vi "S4GUI.vi"(7 "Tab ObsEng":enum32{"Obs", "CCD modes", "Guider", "Eng"}(tab)) -> ()   [LabVIEW 2018] (continued)
        # "real"
        # "Inicializar nova comunicação, de acordo\n com valor de TCS mode\n\nServer.Write id (T=6 ou F=12)\nTCS.Init"
        # "Parar a comunciação atual\nServer.End"
        n1486 = event-data() -> ("NewVal"=w2535:bool)  [unwired: 1 in, 5 out]
        n1487 = call-dynamic "Read TCS.lvclass.vi"("error in (no error)"=w2545, "S4GUI in"=w2546) -> ("error out"=w2540:errorcluster, "TCS.lvclass"=w2543:refnum<class "TCS.lvclass">, "S4GUI out"=w2544:refnum<class "S4GUI.lvclass">)  [unwired: 7 in]
        n1488 = call-dynamic "End.vi"("error in (no error)"=w2540, "Server in"=w2543) -> ("error out"=w2539:errorcluster, "Server out"=w2542:refnum<class "TCS.lvclass">)  [unwired: 8 in]
        n1489 = Select(t=u32 6, s=w2535, f=u32 12) -> (s? t:f=w2549:u32)
        n1490 = call-dynamic "Write id.vi"("error in (no error)"=w2539, "id"=w2549, "Server in"=w2542) -> ("error out"=w2538:errorcluster, "Server out"=w2541:refnum<class "TCS.lvclass">)  [unwired: 7 in]
        n1491 = call-dynamic "Initialize.vi"("error in (no error)"=w2538, "TCS in"=w2541) -> ("error out"=w2536:errorcluster, "TCS out"=w2537:refnum<class "TCS.lvclass">)  [unwired: 8 in]
        n1492 = call-dynamic "Write TCS.lvclass.vi"("error in (no error)"=w2536, "TCS.lvclass"=w2537, "S4GUI in"=w2544) -> ("error out"=w2533:errorcluster, "S4GUI out"=w2534:refnum<class "S4GUI.lvclass">)  [unwired: 7 in]
      }
      event "enter password": Value Change {
        n1493 = event-data() -> ("NewVal"=w2550:bool)  [unwired: 1 in]
        n1494 = case shown="True" w2550 {
          tunnel: [w2556 w2558] -> w2554
          tunnel: [w2555 w2557] -> w2553
          tunnel: w2552 -> [w2556 w2571]
          tunnel: w2551 -> [w2555 w2570]
          frame False {
          }
          frame True {
            # "Verifica senha de configuração de CCD do Administrador"
            n1495 = Equal?(x="password", y="camerasetup") -> (x = y?=w2568:bool)
            n1496 = call-dynamic "Write mode Adm.vi"("error in (no error)"=w2570, "mode Adm"=w2568, "S4GUI in"=w2571) -> ("error out"=w2559:errorcluster, "S4GUI out"=w2560:refnum<class "S4GUI.lvclass">)  [unwired: 7 in]
            n1497 = call-dynamic "Read mode Adm.vi"("error in (no error)"=w2559, "S4GUI in"=w2560) -> ("error out"=w2566:errorcluster, "mode Adm"=w2563:bool, "S4GUI out"=w2565:refnum<class "S4GUI.lvclass">)  [unwired: 7 in]
            n1498 = Select(t="Eng/Camera tab: password OK clicked successful" ("User Event"), s=w2563, f="Eng/Camera tab: password OK clicked with wrong input" ("User Event")) -> (s? t:f=w2564:string)
            n1499 = call-dynamic "Write User Event.vi"("error in (no error)"=w2566, "User Event"=w2564, "S4GUI in"=w2565) -> ("error out"=w2557:errorcluster, "S4GUI out"=w2558:refnum<class "S4GUI.lvclass">)  [unwired: 7 in]
          }
        }
      }
      event "enter password 2": Value Change {
        # "Verificação de senha na aba \"CCD modes\""
        n1500 = event-data() -> ("NewVal"=w2572:bool)  [unwired: 1 in]
        n1501 = case shown="True" w2572 {
          tunnel: [w2578 w2588] -> w2576
          tunnel: [w2577 w2587] -> w2575
          tunnel: w2574 -> [w2578 w2593]
          tunnel: w2573 -> [w2577 w2592]
          frame False {
          }
          frame True {
            # "Verifica senha de configuração de CCD do Administrador"
            n1502 = Equal?(x="password 2", y="ccdmodessetup") -> (x = y?=w2590:bool)
            n1503 = call-dynamic "Write mode Adm.vi"("error in (no error)"=w2592, "mode Adm"=w2590, "S4GUI in"=w2593) -> ("error out"=w2585:errorcluster, "S4GUI out"=w2586:refnum<class "S4GUI.lvclass">)  [unwired: 7 in]
            n1504 = call-dynamic "Read mode Adm.vi"("error in (no error)"=w2585, "S4GUI in"=w2586) -> ("error out"=w2583:errorcluster, "mode Adm"=w2580:bool, "S4GUI out"=w2584:refnum<class "S4GUI.lvclass">)  [unwired: 7 in]
            n1505 = Select(t="CCD mode tab: password OK clicked successful" ("User Event"), s=w2580, f="CCD mode tab: password OK clicked with wrong input" ("User Event")) -> (s? t:f=w2581:string)
            n1506 = call-dynamic "Write User Event.vi"("error in (no error)"=w2583, "User Event"=w2581, "S4GUI in"=w2584) -> ("error out"=w2587:errorcluster, "S4GUI out"=w2588:refnum<class "S4GUI.lvclass">)  [unwired: 7 in]
          }
        }
      }
      event "Tab ObsEng": Value Change {
        n1507 = event-data() -> ("NewVal"=w2594:enum32{"Obs", "CCD modes", "Guider", "Eng"})  [unwired: 1 in]
        n1508 = case shown="Default" w2594 {
          tunnel: [w2608 w2760 w2771] -> w2598
          tunnel: [w2610 w2758 w2769] -> w2597
          tunnel: w2596 -> [w2605 w2766 w2775]
          tunnel: w2595 -> [w2604 w2657 w2770]
          frame "CCD modes" {
            # "Sinaliza que não há requisição de SET CCD mode"
            # "Entrou na aba \"CCD modes\", ajusta para modo usuário normal..."
            n1509 = call-dynamic "Read TabAcqType index.vi"("error in (no error)"=w2604, "S4GUI in"=w2605) -> ("error out"=w2603:errorcluster, "TabAcqType index"=w2601:u32, "S4GUI out"=w2602:refnum<class "S4GUI.lvclass">)  [unwired: 7 in]
            n1510 = case shown="4" w2601 {
              tunnel: w2603 -> [w2640 w2645]
              tunnel: [w2639 w2644] -> w2606
              tunnel: [w2638 w2643] -> w2600
              tunnel: [FALSE ("Visible") TRUE ("Visible")] -> w2599
              frame 0, Default {
                n1511 = local read "Frame Transfer"() -> (w2638:enum16{"OFF", "ON"})
                n1512 = property on="Frame Transfer" class="Enum (strict)"(error in=w2640, "DisabledEnum"=T12."Enabled" ("Disabled")) -> (error out=w2639:errorcluster)  [unwired: 1 in, 1 out]
              }
              frame 4 {
                w2643 = enum16{"OFF", "ON"}."OFF" ("Frame Transfer")
                n1513 = property on="Frame Transfer" class="Enum (strict)"(error in=w2645, "DisabledEnum"=T12."Disabled and Grayed Out" ("Disabled"), "Value"=w2643) -> (error out=w2644:errorcluster)  [unwired: 1 in, 1 out]
              }
            }
            n1514 = property on="FT warning" class="Str"("Caption.Visible"=w2599) -> ()  [unwired: 2 in, 2 out]
            n1515 = call-dynamic "Write mode Adm.vi"("error in (no error)"=w2606, "mode Adm"=FALSE, "S4GUI in"=w2602) -> ("error out"=w2632:errorcluster, "S4GUI out"=w2634:refnum<class "S4GUI.lvclass">)  [unwired: 7 in]
            n1516 = local write "password 2"("" ("password")) -> ()
            n1517 = call-dynamic "Write SET request.vi"("error in (no error)"=w2632, "SET request"=FALSE, "S4GUI in"=w2634) -> ("error out"=w2631:errorcluster, "S4GUI out"=w2633:refnum<class "S4GUI.lvclass">)  [unwired: 7 in]
            n1518 = disable-structure shown="Disabled" {
              frame Disabled {
                n1519 = flat-sequence {
                  tunnel: _ -> [w2653]
                  tunnel: [w2653] -> _
                  frame #0 {
                    n1520 = local read "AQM"() -> (w2650:T4)
                    n1521 = Less Or Equal?(x=w2650, y=T4."NORMAL FAINT: Conventional; 1 MHz; Gain 2") -> (x <= y?=w2649:bool)
                    n1522 = Select(t=w2650, s=w2649, f=T4."SLOW BRIGHT: Conventional; 0.1 MHz; Gain 1" ("y")) -> (s? t:f=w2651:T4)
                    n1523 = local write "EM Gain"(u16 2 ("EM Gain")) -> ()
                    n1524 = local write "AQM"(w2651) -> ()
                  }
                }
              }
              frame Enabled {
              }
            }
            n1525 = flat-sequence {
              tunnel: w2631 -> [w2656]
              tunnel: [w2656] -> w2617
              tunnel: [w2655] -> w2614
              tunnel: [w2654] -> w2615
              frame #0 {
                w2654 = u16 2 ("EM Gain")
                w2655 = T4."NORMAL FAINT: Conventional; 1 MHz; Gain 2" ("AQM")
                n1526 = local write "EM Gain"(w2654) -> ()
                n1527 = local write "AQM"(w2655) -> ()
              }
            }
            n1528 = call-dynamic "Read CCD mode.vi"("error in (no error)"=w2617, "S4GUI in"=w2633) -> ("error out"=w2622:errorcluster, "CCD mode"=w2620:T30, "S4GUI out"=w2619:refnum<class "S4GUI.lvclass">)  [unwired: 7 in]
            n1529 = local read "SZM"() -> (w2616:T3)
            n1530 = Bundle By Name(cluster=w2620, "FTM"=w2600, "SZM"=w2616, "EM gain"=w2615, "AQM"=w2614) -> (w2621:T30)
            n1531 = call-dynamic "Write CCD mode.vi"("error in (no error)"=w2622, "CCD mode"=w2621, "S4GUI in"=w2619) -> ("error out"=w2624:errorcluster, "S4GUI out"=w2623:refnum<class "S4GUI.lvclass">)  [unwired: 7 in]
            n1532 = call-dynamic "LoadCCDmode.vi"("error in (no error)"=w2624, "S4GUI in"=w2623) -> ("error out"=w2626:errorcluster, "S4GUI out"=w2625:refnum<class "S4GUI.lvclass">)  [unwired: 8 in]
            n1533 = call-dynamic "Read Parameters CCD modes.vi"("error in (no error)"=w2626, "S4GUI in"=w2625) -> ("error out"=w2629:errorcluster, "Parameters CCD modes"=w2618:T5, "S4GUI out"=w2627:refnum<class "S4GUI.lvclass">)  [unwired: 7 in]
            n1534 = local write "Parameters CCD modes"(w2618) -> ()
            n1535 = call-dynamic "Read InfoCCDmode.vi"("error in (no error)"=w2629, "S4GUI in"=w2627) -> ("error out"=w2612:errorcluster, "InfoCCDmode"=w2628:T2, "S4GUI out"=w2613:refnum<class "S4GUI.lvclass">)  [unwired: 7 in]
            n1536 = local write "InfoCCDmode"(w2628) -> ()
            n1537 = call-dynamic "CalcTemp.vi"("error in (no error)"=w2612, "S4GUI in"=w2613) -> ("error out"=w2611:errorcluster, "S4GUI out"=w2609:refnum<class "S4GUI.lvclass">)  [unwired: 8 in]
            n1538 = call-dynamic "Read Prev Temp.vi"("error in (no error)"=w2611, "S4GUI in"=w2609) -> ("error out"=w2610:errorcluster, "Prev Temp"=w2607:dbl, "S4GUI out"=w2608:refnum<class "S4GUI.lvclass">)  [unwired: 7 in]
            n1539 = local write "Preview Temp."(w2607) -> ()
          }
          frame "Eng" {
            w2764 = T12."Disabled and Grayed Out" ("Disabled")
            # "Desabilita os botões SET."
            # "Entrou na aba  \"Eng\", ajusta para modo usuário normal..."
            n1540 = local write "password"("" ("password")) -> ()
            n1541 = call-dynamic "Write mode Adm.vi"("error in (no error)"=w2657, "mode Adm"=FALSE, "S4GUI in"=w2766) -> ("error out"=w2759:errorcluster, "S4GUI out"=w2762:refnum<class "S4GUI.lvclass">)  [unwired: 7 in]
            n1542 = property on="Set from Input ch1" class="Bool"("DisabledEnum"=w2764) -> ()  [unwired: 2 in, 2 out]
            n1543 = property on="Set from Input ch3" class="Bool"("DisabledEnum"=w2764) -> ()  [unwired: 2 in, 2 out]
            n1544 = property on="Set from Input ch2" class="Bool"("DisabledEnum"=w2764) -> ()  [unwired: 2 in, 2 out]
            n1545 = property on="Set from Input ch4" class="Bool"("DisabledEnum"=w2764) -> ()  [unwired: 2 in, 2 out]
            n1546 = local read "TARGET NAME WPSEL"() -> (w2715:enum16{"NONE", "OFF", "L/2", "L/4"})
            n1547 = call "Read Instrument.lvclass.vi"("error in (no error)"=w2759, "S4ACS_GUI in"=w2762) -> ("error out"=w2740:errorcluster, "Instrument.lvclass"=w2757:refnum<class "Instrument.lvclass">, "S4ACS_GUI out"=w2761:refnum<class "S4GUI.lvclass">)  [unwired: 7 in]
            n1548 = local read "TARGET NAME CALW"() -> (w2705:T9)
            n1549 = property on="TARGET NAME WPSEL" class="Enum (strict)"() -> ("RingText.Text"=w2713:string)  [unwired: 2 in, 2 out]
            n1550 = call "Read WPSEL.vi"("error in (no error)"=w2740, "Instrument in"=w2757) -> ("error out"=w2755:errorcluster, "Opt_Selector.lvclass"=w2753:refnum<class "Opt_Selector.lvclass">, "Instrument out"=w2756:refnum<class "Instrument.lvclass">)  [unwired: 7 in]
            n1551 = Build Array(-1.0 ("element"), 80.0 ("element"), 0.0 ("element"), 160.0 ("element")) -> (w2716:dbl[])
            n1552 = property on="TARGET NAME CALW" class="Enum (strict)"() -> ("RingText.Text"=w2704:string)  [unwired: 2 in, 2 out]
            n1553 = Build Array(-1.0 ("element"), 0.0 ("element"), 72.0 ("element"), 144.0 ("element"), 216.0 ("element"), 288.0 ("element")) -> (w2708:dbl[])
            n1554 = Index Array "Index Array"(array=w2716, index=w2715) -> (element=w2714:dbl)
            n1555 = call "Write target name.vi"("error in (no error)"=w2755, "target name"=w2713, "Optics in"=w2753) -> ("error out"=w2754:errorcluster, "Optics out"=w2752:refnum<class "Opt_Selector.lvclass">)  [unwired: 7 in]
            n1556 = Index Array(array=w2708, index=w2705) -> (element=w2703:dbl)
            n1557 = call "Write target.vi"("error in (no error)"=w2754, "target"=w2714, "Optics in"=w2752) -> ("error out"=w2750:errorcluster, "Optics out"=w2751:refnum<class "Opt_Selector.lvclass">)  [unwired: 7 in]
            n1558 = call "Write WPSEL.vi"("error in (no error)"=w2750, "Opt_Selector.lvclass"=w2751, "Instrument in"=w2756) -> ("error out"=w2749:errorcluster, "Instrument out"=w2748:refnum<class "Instrument.lvclass">)  [unwired: 7 in]
            n1559 = call "Read CALW.vi"("error in (no error)"=w2749, "Instrument in"=w2748) -> ("error out"=w2746:errorcluster, "Opt_Selector.lvclass"=w2744:refnum<class "Opt_Selector.lvclass">, "Instrument out"=w2741:refnum<class "Instrument.lvclass">)  [unwired: 7 in]
            n1560 = call "Write target name.vi"("error in (no error)"=w2746, "target name"=w2704, "Optics in"=w2744) -> ("error out"=w2747:errorcluster, "Optics out"=w2743:refnum<class "Opt_Selector.lvclass">)  [unwired: 7 in]
            n1561 = call "Write target.vi"("error in (no error)"=w2747, "target"=w2703, "Optics in"=w2743) -> ("error out"=w2745:errorcluster, "Optics out"=w2742:refnum<class "Opt_Selector.lvclass">)  [unwired: 7 in]
            n1562 = local read "TARGET NAME ASEL"() -> (w2697:enum16{"NONE", "OFF", "ON"})
            n1563 = call "Write CALW.vi"("error in (no error)"=w2745, "Opt_Selector.lvclass"=w2742, "Instrument in"=w2741) -> ("error out"=w2737:errorcluster, "Instrument out"=w2738:refnum<class "Instrument.lvclass">)  [unwired: 7 in]
            n1564 = property on="TARGET NAME ASEL" class="Enum (strict)"() -> ("RingText.Text"=w2698:string)  [unwired: 2 in, 2 out]
            n1565 = Build Array(-1.0 ("element"), 0.0 ("element"), 30.0 ("element")) -> (w2699:dbl[])
            n1566 = Index Array(array=w2699, index=w2697) -> (element=w2696:dbl)
            n1567 = call "Read ASEL.vi"("error in (no error)"=w2737, "Instrument in"=w2738) -> ("error out"=w2736:errorcluster, "Opt_Selector.lvclass"=w2734:refnum<class "Opt_Selector.lvclass">, "Instrument out"=w2731:refnum<class "Instrument.lvclass">)  [unwired: 7 in]
            n1568 = call "Write target name.vi"("error in (no error)"=w2736, "target name"=w2698, "Optics in"=w2734) -> ("error out"=w2739:errorcluster, "Optics out"=w2733:refnum<class "Opt_Selector.lvclass">)  [unwired: 7 in]
            n1569 = call "Write target.vi"("error in (no error)"=w2739, "target"=w2696, "Optics in"=w2733) -> ("error out"=w2735:errorcluster, "Optics out"=w2732:refnum<class "Opt_Selector.lvclass">)  [unwired: 7 in]
            n1570 = call "Write ASEL.vi"("error in (no error)"=w2735, "Opt_Selector.lvclass"=w2732, "Instrument in"=w2731) -> ("error out"=w2730:errorcluster, "Instrument out"=w2729:refnum<class "Instrument.lvclass">)  [unwired: 7 in]
            n1571 = local read "GMIR_target"() -> (w2690:dbl)
            n1572 = local read "GFOC_target"() -> (w2691:dbl)
            n1573 = call "Read GFOC.vi"("error in (no error)"=w2730, "Instrument in"=w2729) -> ("error out"=w2694:errorcluster, "Opt_Continuous.lvclass"=w2695:refnum<class "Opt_Continuous.lvclass">, "Instrument out"=w2726:refnum<class "Instrument.lvclass">)  [unwired: 7 in]
            n1574 = call "Write target.vi"("error in (no error)"=w2694, "target"=w2691, "Optics in"=w2695) -> ("error out"=w2728:errorcluster, "Optics out"=w2725:refnum<class "Opt_Continuous.lvclass">)  [unwired: 7 in]
            n1575 = call "Write GFOC.vi"("error in (no error)"=w2728, "Opt_Continuous.lvclass"=w2725, "Instrument in"=w2726) -> ("error out"=w2727:errorcluster, "Instrument out"=w2724:refnum<class "Instrument.lvclass">)  [unwired: 7 in]
            n1576 = call "Read GMIR.vi"("error in (no error)"=w2727, "Instrument in"=w2724) -> ("error out"=w2692:errorcluster, "Opt_Continuous.lvclass"=w2693:refnum<class "Opt_Continuous.lvclass">, "Instrument out"=w2723:refnum<class "Instrument.lvclass">)  [unwired: 7 in]
            n1577 = call "Write target.vi"("error in (no error)"=w2692, "target"=w2690, "Optics in"=w2693) -> ("error out"=w2721:errorcluster, "Optics out"=w2722:refnum<class "Opt_Continuous.lvclass">)  [unwired: 7 in]
            n1578 = local read "TARGET NAME WPROT"() -> (w2659:T10)
            n1579 = call "Write GMIR.vi"("error in (no error)"=w2721, "Opt_Continuous.lvclass"=w2722, "Instrument in"=w2723) -> ("error out"=w2686:errorcluster, "Instrument out"=w2685:refnum<class "Instrument.lvclass">)  [unwired: 7 in]
            n1580 = property on="TARGET NAME WPROT" class="Enum (strict)"() -> ("RingText.Text"=w2658:string)  [unwired: 2 in, 2 out]
            n1581 = call "Read WPROT.vi"("error in (no error)"=w2686, "Instrument in"=w2685) -> ("error out"=w2683:errorcluster, "Opt_Selector.lvclass"=w2687:refnum<class "Opt_Selector.lvclass">, "Instrument out"=w2684:refnum<class "Instrument.lvclass">)  [unwired: 7 in]
            n1582 = Build Array(-1.0 ("element"), 0.0 ("element"), 22.5 ("element"), 45.0 ("element"), 67.5 ("element"), 90.0 ("element"), 112.5 ("element"), 135.0 ("element"), 157.5 ("element"), 180.0 ("element"), 202.5 ("element"), 225.0 ("element"), 247.5 ("element"), 270.0 ("element"), 292.5 ("element"), 315.0 ("element"), 337.5 ("element")) -> (w2672:dbl[])
            n1583 = Index Array(array=w2672, index=w2659) -> (element=w2660:dbl)
            n1584 = call "Write target name.vi"("error in (no error)"=w2683, "target name"=w2658, "Optics in"=w2687) -> ("error out"=w2682:errorcluster, "Optics out"=w2689:refnum<class "Opt_Selector.lvclass">)  [unwired: 7 in]
            n1585 = call "Write target.vi"("error in (no error)"=w2682, "target"=w2660, "Optics in"=w2689) -> ("error out"=w2681:errorcluster, "Optics out"=w2688:refnum<class "Opt_Selector.lvclass">)  [unwired: 7 in]
            n1586 = call "Write WPROT.vi"("error in (no error)"=w2681, "Opt_Selector.lvclass"=w2688, "Instrument in"=w2684) -> ("error out"=w2679:errorcluster, "Instrument out"=w2680:refnum<class "Instrument.lvclass">)  [unwired: 7 in]
            n1587 = call "Write Instrument.lvclass.vi"("error in (no error)"=w2679, "Instrument.lvclass"=w2680, "S4ACS_GUI in"=w2761) -> ("error out"=w2758:errorcluster, "S4ACS_GUI out"=w2760:refnum<class "S4GUI.lvclass">)  [unwired: 7 in]
          }
          frame Default {
            n1588 = call "Read Instrument.lvclass.vi"("error in (no error)"=w2770, "S4ACS_GUI in"=w2775) -> ("error out"=w2769:errorcluster, "Instrument.lvclass"=w2774:refnum<class "Instrument.lvclass">, "S4ACS_GUI out"=w2771:refnum<class "S4GUI.lvclass">)  [unwired: 7 in]
            n1589 = call "Read WPSEL.vi"("Instrument in"=w2774) -> ("Opt_Selector.lvclass"=w2773:refnum<class "Opt_Selector.lvclass">)  [unwired: 8 in, 2 out]
            n1590 = call "Read name_pos.vi"("Optics in"=w2773) -> ("name_pos"=w2772:string)  [unwired: 8 in, 2 out]
            n1591 = case shown="\"OFF\", Default" w2772 {
              tunnel: [w2777 w2779 w2781] -> w2768
              tunnel: ["Lambda/4" ("Ring Text.Text") "Lambda/2" ("Ring Text.Text") "OFF" ("Ring Text.Text")] -> w2767
              frame "L/4" {
                w2777 = u16 2 items=["OFF", "Lambda/2", "Lambda/4"] ("Lambda Selector")
              }
              frame "L/2" {
                w2779 = u16 1 items=["OFF", "Lambda/2", "Lambda/4"] ("Lambda Selector")
              }
              frame "OFF", Default {
                w2781 = u16 0 items=["OFF", "Lambda/2", "Lambda/4"] ("Lambda Selector")
              }
            }
            n1592 = property on="Lambda Selector" class="Ring (strict)"("Value"=w2768, "RingText.Text"=w2767) -> ()  [unwired: 2 in, 2 out]
          }
        }
      }
      event "S4ICS protocol": Value Change {
        # "2024-04-04: Não se usa mais o ID para configurar a comunicação..."
        # "TCP-IP"
        # "ZeroMQ"
        # "Inicializar nova comunicação, de acordo\n com valor de S4ICS mode\n\nServer.Write id (T=13 ou F=5)\nInstrument.Init"
        # "Parar a comunciação atual\nServer.End"
        n1593 = event-data() -> ("NewVal"=w2784:bool)  [unwired: 1 in, 5 out]
        n1594 = call "Read Instrument.lvclass.vi"("error in (no error)"=w2794, "S4ACS_GUI in"=w2795) -> ("error out"=w2789:errorcluster, "Instrument.lvclass"=w2792:refnum<class "Instrument.lvclass">, "S4ACS_GUI out"=w2793:refnum<class "S4GUI.lvclass">)  [unwired: 7 in]
        n1595 = call-dynamic "End.vi"("error in (no error)"=w2789, "Server in"=w2792) -> ("error out"=w2788:errorcluster, "Server out"=w2791:refnum<class "Instrument.lvclass">)  [unwired: 8 in]
        n1596 = Select(t=u32 13, s=w2784, f=u32 5) -> (s? t:f=w2798:u32)
        n1597 = call-dynamic "Write id.vi"("error in (no error)"=w2788, "id"=w2798, "Server in"=w2791) -> ("error out"=w2787:errorcluster, "Server out"=w2790:refnum<class "Instrument.lvclass">)  [unwired: 7 in]
        n1598 = call-dynamic "Initialize.vi"("error in (no error)"=w2787, "Instrument in"=w2790) -> ("error out"=w2785:errorcluster, "Instrument out"=w2786:refnum<class "Instrument.lvclass">)  [unwired: 8 in]
        n1599 = call "Write Instrument.lvclass.vi"("error in (no error)"=w2785, "Instrument.lvclass"=w2786, "S4ACS_GUI in"=w2793) -> ("error out"=w2782:errorcluster, "S4ACS_GUI out"=w2783:refnum<class "S4GUI.lvclass">)  [unwired: 7 in]
      }
      event "Set from Input ch1": Value Change {
        # "ACS"
        # "GUI"
        # "EM_MODE = E.M."
        # "Readou Rate:\n30         0\n20         1     \n10         2\n1           3"
        # "EM_MODE = Conv"
        # "Readou Rate:\n1         0\n0.1      1"
        # "Readou Rate:\n1         0\n0.1      1     \n10       2\n20       3\n30       4"
        n1600 = event-data() -> ()  [unwired: 1 in, 6 out]
        n1601 = local read "Input Cluster"() -> (w2823:T8)
        n1602 = Unbundle By Name(w2823) -> ("Parameters"=w2822:T5)
        n1603 = Unbundle By Name(w2822) -> ("Image \nInitial Line"=w2850:u16, "Image\nInitial Column"=w2849:u16, "Image\nFinal Line"=w2848:u16, "Image\nFInal Column"=w2847:u16, "Vertical\nBinning"=w2846:u16, "Horizontal\nBinning"=w2845:u16, "Pre-amplification\nGain"=w2844:u8, "CCD\nEM Gain"=w2843:u16, "Readout\nRate"=w2842:u8, "Shutter\nOpenning Time"=w2841:i32, "Shutter\nClosing Time"=w2840:i32, "Vertical\nShift Speed"=w2839:u8, "Read\nMode"=w2838:u8, "Vertical\nClock Voltage"=w2837:u8, "A/D \nChannel"=w2836:u32, "Shutter\nMode"=w2835:u16, "Shutter\nTTL"=w2834:u16, "Trigger\nMode"=w2833:u16, "Frame\nTransfer"=w2814:bool, "Acquisition\nMode"=w2832:u8, "CCD \nEM Mode"=w2831:u8)
        n1604 = call-dynamic "Write User Event.vi"("error in (no error)"=w2802, "User Event"="SET CCD CONFIG CHANNEL1 ", "S4GUI in"=w2803) -> ("error out"=w2800:errorcluster, "S4GUI out"=w2801:refnum<class "S4GUI.lvclass">)  [unwired: 7 in]
        n1605 = call-dynamic "Read AcquisitionA.vi"("error in (no error)"=w2800, "S4ACS_GUI in"=w2801) -> ("error out"=w2866:errorcluster, "Acquisition.lvclass"=w2869:refnum<class "Acquisition.lvclass">, "S4ACS_GUI out"=w2870:refnum<class "S4GUI.lvclass">)  [unwired: 7 in]
        n1606 = call-dynamic "Read Channel.vi"("error in (no error)"=w2866, "Acquisition in"=w2869) -> ("error out"=w2865:errorcluster, "Channel.lvclass"=w2867:refnum<class "Channel.lvclass">, "Acquisition out"=w2868:refnum<class "Acquisition.lvclass">)  [unwired: 7 in]
        n1607 = call-dynamic "Read Interface.vi"("error in (no error)"=w2865, "Channel in"=w2867) -> ("error out"=w2813:errorcluster, "Interface.lvclass"=w2815:refnum<class "Interface.lvclass">, "Channel out"=w2810:refnum<class "Channel.lvclass">)  [unwired: 7 in]
        n1608 = call-dynamic "Write PREV_FT.vi"("error in (no error)"=w2813, "PREV_FT"=w2814, "Interface in"=w2815) -> ("error out"=w2812:errorcluster, "Interface out"=w2811:refnum<class "Interface.lvclass">)  [unwired: 7 in]
        n1609 = call-dynamic "Read target cluster.vi"("error in (no error)"=w2812, "Channel in"=w2810) -> ("error out"=w2808:errorcluster, "target cluster"=w2806:T31, "Channel out"=w2807:refnum<class "Channel.lvclass">)  [unwired: 7 in]
        n1610 = Bundle By Name(cluster=w2806, "INITIAL_LINE"=w2850, "INITIAL_COLUMN"=w2849, "FINAL_LINE"=w2848, "FINAL_COLUMN"=w2847, "VBIN"=w2846, "HBIN"=w2845, "PREAMP"=w2844, "EM_GAIN"=w2843, "READOUT_RATE"=w2842, "SHUTTER_OPENING_TIME"=w2841, "SHUTTER_CLOSING_TIME"=w2840, "VERTICAL_SHIFT_SPEED"=w2839, "READ_MODE"=w2838, "VERTICAL_CLOCK_VOLTAGE"=w2837, "AD_CHANNEL"=w2836, "SHUTTER_MODE"=w2835, "SHUTTER_TTL"=w2834, "TRIGGER_MODE"=w2833, "FRAME_TRANSFER"=w2814, "ACQUISITION_MODE"=w2832, "EM_MODE"=w2831) -> (w2805:T31)
        n1611 = call-dynamic "Write target cluster.vi"("error in (no error)"=w2808, "target cluster"=w2805, "Channel in"=w2807) -> ("error out"=w2804:errorcluster, "Channel out"=w2809:refnum<class "Channel.lvclass">)  [unwired: 7 in]
        n1612 = Flatten To String(anything=w2805, error in (no error)=w2804) -> (data string=w2854:string, error out=w2853:errorcluster)  [unwired: 2 in, 1 out]
        n1613 = call "Write flatted cluster.vi"("error in (no error)"=w2853, "flatted cluster"=w2854, "Interface in"=w2811) -> ("error out"=w2852:errorcluster, "Interface out"=w2851:refnum<class "Interface.lvclass">)  [unwired: 7 in]
        n1614 = call-dynamic "Write Interface.vi"("error in (no error)"=w2852, "Interface.lvclass"=w2851, "Channel in"=w2809) -> ("error out"=w2826:errorcluster, "Channel out"=w2829:refnum<class "Channel.lvclass">)  [unwired: 7 in]
        n1615 = call "Write section_name.vi"("error in (no error)"=w2826, "section_name"="CCD_ACS1", "Channel in"=w2829) -> ("error out"=w2825:errorcluster, "Channel out"=w2828:refnum<class "Channel.lvclass">)  [unwired: 7 in]
        n1616 = call-dynamic "save config.vi"("error in (no error)"=w2825, "file config"="lastsaved.cfg", "Channel in"=w2828) -> ("error out"=w2824:errorcluster, "Channel out"=w2827:refnum<class "Channel.lvclass">)  [unwired: 7 in]
        n1617 = call-dynamic "Read State Machine.vi"("error in (no error)"=w2824, "Device in"=w2827) -> ("error out"=w2861:errorcluster, "State Machine.lvclass"=w2863:refnum<class "State Machine.lvclass">, "Device out"=w2864:refnum<class "Channel.lvclass">)  [unwired: 7 in]
        n1618 = call-dynamic "Write State.vi"("error in (no error)"=w2861, "State"=60, "State Machine in"=w2863) -> ("error out"=w2860:errorcluster, "State Machine out"=w2862:refnum<class "State Machine.lvclass">)  [unwired: 7 in]
        n1619 = call-dynamic "Write State Machine.vi"("error in (no error)"=w2860, "State Machine.lvclass"=w2862, "Device in"=w2864) -> ("error out"=w2857:errorcluster, "Device out"=w2858:refnum<class "Channel.lvclass">)  [unwired: 7 in]
        n1620 = call-dynamic "Write Channel.vi"("error in (no error)"=w2857, "Channel.lvclass"=w2858, "Acquisition in"=w2868) -> ("error out"=w2856:errorcluster, "Acquisition out"=w2855:refnum<class "Acquisition.lvclass">)  [unwired: 7 in]
        n1621 = call-dynamic "Write AcquisitionA.vi"("error in (no error)"=w2856, "Acquisition.lvclass"=w2855, "S4ACS_GUI in"=w2870) -> ("error out"=w2817:errorcluster, "S4ACS_GUI out"=w2818:refnum<class "S4GUI.lvclass">)  [unwired: 7 in]
        n1622 = call "Write cfg file.vi"("error in (no error)"=w2817, "cfg file"="lastsaved.cfg", "S4ACS_GUI in"=w2818) -> ("error out"=w2820:errorcluster, "S4ACS_GUI out"=w2821:refnum<class "S4GUI.lvclass">)  [unwired: 7 in]
      }
      event "Input Cluster.Parameters.CCD \nEM Mode": Value Change {
        n1623 = event-data() -> ()  [unwired: 1 in, 6 out]
        n1624 = local read "Input Cluster"() -> (w2885:T8)
        n1625 = Unbundle By Name(w2885) -> ("Parameters"=w2886:T5)
        n1626 = Unbundle By Name(w2886) -> ("Readout\nRate"=→"Readout\nRate":u8, "CCD \nEM Mode"=w2880:u8)
        n1627 = case shown="0, Default" w2880 {
          tunnel: [string[] ["30 MHz", "20 MHz", "10 MHz", "1 MHz"] ("Strings []") string[] ["1 MHz", "0.1 MHz"] ("Strings []")] -> w2879
          tunnel: [u8 3 u8 0] -> w2878
          frame 0, Default {
          }
          frame 1 {
          }
        }
        n1628 = local read "Cameras Cluster"() -> (w2873:T7)
        n1629 = flat-sequence {
          tunnel: w2878 -> [w2888]
          tunnel: w2879 -> [w2887]
          tunnel: w2880 -> [w2889]
          tunnel: [w2889] -> w2877
          tunnel: [w2888] -> w2875
          tunnel: w2886 -> [w2895]
          tunnel: [w2894] -> w2884
          tunnel: w2877 -> [w2890]
          tunnel: w2875 -> [w2891]
          tunnel: w2874 -> [w2893]
          tunnel: [w2892] -> w2872
          frame #0 {
            n1630 = property on="Readout\nRate" class="Ring (strict)"("Strings []"=w2887) -> ()  [unwired: 2 in, 2 out]
            n1631 = property on="Readout Rate" class="Ring (strict)"("Strings []"=w2887) -> ()  [unwired: 2 in, 2 out]
            n1632 = property on="Readout Rate 4" class="Ring (strict)"("Strings []"=w2887) -> ()  [unwired: 2 in, 2 out]
            n1633 = property on="Readout Rate 2" class="Ring (strict)"("Strings []"=w2887) -> ()  [unwired: 2 in, 2 out]
            n1634 = property on="Readout Rate 3" class="Ring (strict)"("Strings []"=w2887) -> ()  [unwired: 2 in, 2 out]
          }
          frame #1 {
            n1635 = Bundle By Name(cluster=w2893, "Readout Rate"=w2891, "Read Mode"=w2890) -> (w2892:T32)
            n1636 = Bundle By Name(cluster=w2895, "Readout\nRate"=w2891, "CCD \nEM Mode"=w2890) -> (w2894:T5)
          }
        }
        n1637 = Unbundle By Name(w2873) -> ("Current Configuration"=w2874:T32)
        n1638 = Bundle By Name(cluster=w2885, "Parameters"=w2884) -> (w2883:T8)
        n1639 = local write "Input Cluster"(w2883) -> ()
        n1640 = Bundle By Name(cluster=w2873, "Current Configuration"=w2872) -> (w2871:T7)
        n1641 = local write "Cameras Cluster"(w2871) -> ()
      }
      event "Set from Input ch2": Value Change {
        n1642 = event-data() -> ()  [unwired: 1 in, 6 out]
        n1643 = local read "Input Cluster"() -> (w2924:T8)
        n1644 = Unbundle By Name(w2924) -> ("Parameters"=w2923:T5)
        n1645 = call-dynamic "Write User Event.vi"("error in (no error)"=w2902, "User Event"="SET CCD CONFIG CHANNEL2 ", "S4GUI in"=w2903) -> ("error out"=w2900:errorcluster, "S4GUI out"=w2901:refnum<class "S4GUI.lvclass">)  [unwired: 7 in]
        n1646 = Unbundle By Name(w2923) -> ("Image \nInitial Line"=w2951:u16, "Image\nInitial Column"=w2950:u16, "Image\nFinal Line"=w2949:u16, "Image\nFInal Column"=w2948:u16, "Vertical\nBinning"=w2947:u16, "Horizontal\nBinning"=w2946:u16, "Pre-amplification\nGain"=w2945:u8, "CCD\nEM Gain"=w2944:u16, "Readout\nRate"=w2943:u8, "Shutter\nOpenning Time"=w2942:i32, "Shutter\nClosing Time"=w2941:i32, "Vertical\nShift Speed"=w2940:u8, "Read\nMode"=w2939:u8, "Vertical\nClock Voltage"=w2938:u8, "A/D \nChannel"=w2937:u32, "Shutter\nMode"=w2936:u16, "Shutter\nTTL"=w2935:u16, "Trigger\nMode"=w2934:u16, "Frame\nTransfer"=w2914:bool, "Acquisition\nMode"=w2933:u8, "CCD \nEM Mode"=w2932:u8)
        n1647 = call "Read AcquisitionB.vi"("error in (no error)"=w2900, "S4ACS_GUI in"=w2901) -> ("error out"=w2967:errorcluster, "Acquisition.lvclass"=w2970:refnum<class "Acquisition.lvclass">, "S4ACS_GUI out"=w2971:refnum<class "S4GUI.lvclass">)  [unwired: 7 in]
        n1648 = call-dynamic "Read Channel.vi"("error in (no error)"=w2967, "Acquisition in"=w2970) -> ("error out"=w2966:errorcluster, "Channel.lvclass"=w2968:refnum<class "Channel.lvclass">, "Acquisition out"=w2969:refnum<class "Acquisition.lvclass">)  [unwired: 7 in]
        n1649 = call-dynamic "Read Interface.vi"("error in (no error)"=w2966, "Channel in"=w2968) -> ("error out"=w2915:errorcluster, "Interface.lvclass"=w2916:refnum<class "Interface.lvclass">, "Channel out"=w2911:refnum<class "Channel.lvclass">)  [unwired: 7 in]
        n1650 = call-dynamic "Write PREV_FT.vi"("error in (no error)"=w2915, "PREV_FT"=w2914, "Interface in"=w2916) -> ("error out"=w2908:errorcluster, "Interface out"=w2906:refnum<class "Interface.lvclass">)  [unwired: 7 in]
        n1651 = call-dynamic "Read target cluster.vi"("error in (no error)"=w2908, "Channel in"=w2911) -> ("error out"=w2913:errorcluster, "target cluster"=w2910:T31, "Channel out"=w2912:refnum<class "Channel.lvclass">)  [unwired: 7 in]
        n1652 = Bundle By Name(cluster=w2910, "INITIAL_LINE"=w2951, "INITIAL_COLUMN"=w2950, "FINAL_LINE"=w2949, "FINAL_COLUMN"=w2948, "VBIN"=w2947, "HBIN"=w2946, "PREAMP"=w2945, "EM_GAIN"=w2944, "READOUT_RATE"=w2943, "SHUTTER_OPENING_TIME"=w2942, "SHUTTER_CLOSING_TIME"=w2941, "VERTICAL_SHIFT_SPEED"=w2940, "READ_MODE"=w2939, "VERTICAL_CLOCK_VOLTAGE"=w2938, "AD_CHANNEL"=w2937, "SHUTTER_MODE"=w2936, "SHUTTER_TTL"=w2935, "TRIGGER_MODE"=w2934, "FRAME_TRANSFER"=w2914, "ACQUISITION_MODE"=w2933, "EM_MODE"=w2932) -> (w2909:T31)
        n1653 = call-dynamic "Write target cluster.vi"("error in (no error)"=w2913, "target cluster"=w2909, "Channel in"=w2912) -> ("error out"=w2907:errorcluster, "Channel out"=w2905:refnum<class "Channel.lvclass">)  [unwired: 7 in]
        n1654 = Flatten To String(anything=w2909, error in (no error)=w2907) -> (data string=w2955:string, error out=w2954:errorcluster)  [unwired: 2 in, 1 out]
        n1655 = call "Write flatted cluster.vi"("error in (no error)"=w2954, "flatted cluster"=w2955, "Interface in"=w2906) -> ("error out"=w2953:errorcluster, "Interface out"=w2952:refnum<class "Interface.lvclass">)  [unwired: 7 in]
        n1656 = call-dynamic "Write Interface.vi"("error in (no error)"=w2953, "Interface.lvclass"=w2952, "Channel in"=w2905) -> ("error out"=w2927:errorcluster, "Channel out"=w2930:refnum<class "Channel.lvclass">)  [unwired: 7 in]
        n1657 = call "Write section_name.vi"("error in (no error)"=w2927, "section_name"="CCD_ACS2", "Channel in"=w2930) -> ("error out"=w2926:errorcluster, "Channel out"=w2929:refnum<class "Channel.lvclass">)  [unwired: 7 in]
        n1658 = call-dynamic "save config.vi"("error in (no error)"=w2926, "file config"="lastsaved.cfg", "Channel in"=w2929) -> ("error out"=w2925:errorcluster, "Channel out"=w2928:refnum<class "Channel.lvclass">)  [unwired: 7 in]
        n1659 = call-dynamic "Read State Machine.vi"("error in (no error)"=w2925, "Device in"=w2928) -> ("error out"=w2962:errorcluster, "State Machine.lvclass"=w2964:refnum<class "State Machine.lvclass">, "Device out"=w2965:refnum<class "Channel.lvclass">)  [unwired: 7 in]
        n1660 = call-dynamic "Write State.vi"("error in (no error)"=w2962, "State"=60, "State Machine in"=w2964) -> ("error out"=w2961:errorcluster, "State Machine out"=w2963:refnum<class "State Machine.lvclass">)  [unwired: 7 in]
        n1661 = call-dynamic "Write State Machine.vi"("error in (no error)"=w2961, "State Machine.lvclass"=w2963, "Device in"=w2965) -> ("error out"=w2958:errorcluster, "Device out"=w2959:refnum<class "Channel.lvclass">)  [unwired: 7 in]
        n1662 = call-dynamic "Write Channel.vi"("error in (no error)"=w2958, "Channel.lvclass"=w2959, "Acquisition in"=w2969) -> ("error out"=w2957:errorcluster, "Acquisition out"=w2956:refnum<class "Acquisition.lvclass">)  [unwired: 7 in]
        n1663 = call "Write AcquisitionB.vi"("error in (no error)"=w2957, "Acquisition.lvclass"=w2956, "S4ACS_GUI in"=w2971) -> ("error out"=w2917:errorcluster, "S4ACS_GUI out"=w2918:refnum<class "S4GUI.lvclass">)  [unwired: 7 in]
        n1664 = call "Write cfg file.vi"("error in (no error)"=w2917, "cfg file"="lastsaved.cfg", "S4ACS_GUI in"=w2918) -> ("error out"=w2920:errorcluster, "S4ACS_GUI out"=w2921:refnum<class "S4GUI.lvclass">)  [unwired: 7 in]
      }
      event "Set from Input ch3": Value Change {
        n1665 = event-data() -> ()  [unwired: 1 in, 6 out]
        n1666 = local read "Input Cluster"() -> (w2996:T8)
        n1667 = Unbundle By Name(w2996) -> ("Parameters"=w2995:T5)
        n1668 = call-dynamic "Write User Event.vi"("error in (no error)"=w2974, "User Event"="SET CCD CONFIG CHANNEL 3 ", "S4GUI in"=w2975) -> ("error out"=w2972:errorcluster, "S4GUI out"=w2973:refnum<class "S4GUI.lvclass">)  [unwired: 7 in]
        n1669 = Unbundle By Name(w2995) -> ("Image \nInitial Line"=w3023:u16, "Image\nInitial Column"=w3022:u16, "Image\nFinal Line"=w3021:u16, "Image\nFInal Column"=w3020:u16, "Vertical\nBinning"=w3019:u16, "Horizontal\nBinning"=w3018:u16, "Pre-amplification\nGain"=w3017:u8, "CCD\nEM Gain"=w3016:u16, "Readout\nRate"=w3015:u8, "Shutter\nOpenning Time"=w3014:i32, "Shutter\nClosing Time"=w3013:i32, "Vertical\nShift Speed"=w3012:u8, "Read\nMode"=w3011:u8, "Vertical\nClock Voltage"=w3010:u8, "A/D \nChannel"=w3009:u32, "Shutter\nMode"=w3008:u16, "Shutter\nTTL"=w3007:u16, "Trigger\nMode"=w3006:u16, "Frame\nTransfer"=w2986:bool, "Acquisition\nMode"=w3005:u8, "CCD \nEM Mode"=w3004:u8)
        n1670 = call-dynamic "Read AcquisitionC.vi"("error in (no error)"=w2972, "S4ACS_GUI in"=w2973) -> ("error out"=w3039:errorcluster, "Acquisition.lvclass"=w3042:refnum<class "Acquisition.lvclass">, "S4ACS_GUI out"=w3043:refnum<class "S4GUI.lvclass">)  [unwired: 7 in]
        n1671 = call-dynamic "Read Channel.vi"("error in (no error)"=w3039, "Acquisition in"=w3042) -> ("error out"=w3038:errorcluster, "Channel.lvclass"=w3040:refnum<class "Channel.lvclass">, "Acquisition out"=w3041:refnum<class "Acquisition.lvclass">)  [unwired: 7 in]
        n1672 = call-dynamic "Read Interface.vi"("error in (no error)"=w3038, "Channel in"=w3040) -> ("error out"=w2987:errorcluster, "Interface.lvclass"=w2988:refnum<class "Interface.lvclass">, "Channel out"=w2983:refnum<class "Channel.lvclass">)  [unwired: 7 in]
        n1673 = call-dynamic "Write PREV_FT.vi"("error in (no error)"=w2987, "PREV_FT"=w2986, "Interface in"=w2988) -> ("error out"=w2977:errorcluster, "Interface out"=w2984:refnum<class "Interface.lvclass">)  [unwired: 7 in]
        n1674 = call-dynamic "Read target cluster.vi"("error in (no error)"=w2977, "Channel in"=w2983) -> ("error out"=w2985:errorcluster, "target cluster"=w2979:T31, "Channel out"=w2982:refnum<class "Channel.lvclass">)  [unwired: 7 in]
        n1675 = Bundle By Name(cluster=w2979, "INITIAL_LINE"=w3023, "INITIAL_COLUMN"=w3022, "FINAL_LINE"=w3021, "FINAL_COLUMN"=w3020, "VBIN"=w3019, "HBIN"=w3018, "PREAMP"=w3017, "EM_GAIN"=w3016, "READOUT_RATE"=w3015, "SHUTTER_OPENING_TIME"=w3014, "SHUTTER_CLOSING_TIME"=w3013, "VERTICAL_SHIFT_SPEED"=w3012, "READ_MODE"=w3011, "VERTICAL_CLOCK_VOLTAGE"=w3010, "AD_CHANNEL"=w3009, "SHUTTER_MODE"=w3008, "SHUTTER_TTL"=w3007, "TRIGGER_MODE"=w3006, "FRAME_TRANSFER"=w2986, "ACQUISITION_MODE"=w3005, "EM_MODE"=w3004) -> (w2978:T31)
        n1676 = call-dynamic "Write target cluster.vi"("error in (no error)"=w2985, "target cluster"=w2978, "Channel in"=w2982) -> ("error out"=w2980:errorcluster, "Channel out"=w2981:refnum<class "Channel.lvclass">)  [unwired: 7 in]
        n1677 = Flatten To String(anything=w2978, error in (no error)=w2980) -> (data string=w3027:string, error out=w3026:errorcluster)  [unwired: 2 in, 1 out]
        n1678 = call "Write flatted cluster.vi"("error in (no error)"=w3026, "flatted cluster"=w3027, "Interface in"=w2984) -> ("error out"=w3025:errorcluster, "Interface out"=w3024:refnum<class "Interface.lvclass">)  [unwired: 7 in]
        n1679 = call-dynamic "Write Interface.vi"("error in (no error)"=w3025, "Interface.lvclass"=w3024, "Channel in"=w2981) -> ("error out"=w2999:errorcluster, "Channel out"=w3002:refnum<class "Channel.lvclass">)  [unwired: 7 in]
        n1680 = call "Write section_name.vi"("error in (no error)"=w2999, "section_name"="CCD_ACS3", "Channel in"=w3002) -> ("error out"=w2998:errorcluster, "Channel out"=w3001:refnum<class "Channel.lvclass">)  [unwired: 7 in]
        n1681 = call-dynamic "save config.vi"("error in (no error)"=w2998, "file config"="lastsaved.cfg", "Channel in"=w3001) -> ("error out"=w2997:errorcluster, "Channel out"=w3000:refnum<class "Channel.lvclass">)  [unwired: 7 in]
        n1682 = call-dynamic "Read State Machine.vi"("error in (no error)"=w2997, "Device in"=w3000) -> ("error out"=w3034:errorcluster, "State Machine.lvclass"=w3036:refnum<class "State Machine.lvclass">, "Device out"=w3037:refnum<class "Channel.lvclass">)  [unwired: 7 in]
        n1683 = call-dynamic "Write State.vi"("error in (no error)"=w3034, "State"=60, "State Machine in"=w3036) -> ("error out"=w3033:errorcluster, "State Machine out"=w3035:refnum<class "State Machine.lvclass">)  [unwired: 7 in]
        n1684 = call-dynamic "Write State Machine.vi"("error in (no error)"=w3033, "State Machine.lvclass"=w3035, "Device in"=w3037) -> ("error out"=w3030:errorcluster, "Device out"=w3031:refnum<class "Channel.lvclass">)  [unwired: 7 in]
        n1685 = call-dynamic "Write Channel.vi"("error in (no error)"=w3030, "Channel.lvclass"=w3031, "Acquisition in"=w3041) -> ("error out"=w3029:errorcluster, "Acquisition out"=w3028:refnum<class "Acquisition.lvclass">)  [unwired: 7 in]
        n1686 = call-dynamic "Write AcquisitionC.vi"("error in (no error)"=w3029, "Acquisition.lvclass"=w3028, "S4ACS_GUI in"=w3043) -> ("error out"=w2989:errorcluster, "S4ACS_GUI out"=w2990:refnum<class "S4GUI.lvclass">)  [unwired: 7 in]
        n1687 = call "Write cfg file.vi"("error in (no error)"=w2989, "cfg file"="lastsaved.cfg", "S4ACS_GUI in"=w2990) -> ("error out"=w2992:errorcluster, "S4ACS_GUI out"=w2993:refnum<class "S4GUI.lvclass">)  [unwired: 7 in]
      }
      event "Set from Input ch4": Value Change {
        n1688 = event-data() -> ()  [unwired: 1 in, 6 out]
        n1689 = local read "Input Cluster"() -> (w3068:T8)
        n1690 = Unbundle By Name(w3068) -> ("Parameters"=w3067:T5)
        n1691 = call-dynamic "Write User Event.vi"("error in (no error)"=w3047, "User Event"="SET CCD CONFIG CHANNEL4 ", "S4GUI in"=w3046) -> ("error out"=w3044:errorcluster, "S4GUI out"=w3045:refnum<class "S4GUI.lvclass">)  [unwired: 7 in]
        n1692 = Unbundle By Name(w3067) -> ("Image \nInitial Line"=w3095:u16, "Image\nInitial Column"=w3094:u16, "Image\nFinal Line"=w3093:u16, "Image\nFInal Column"=w3092:u16, "Vertical\nBinning"=w3091:u16, "Horizontal\nBinning"=w3090:u16, "Pre-amplification\nGain"=w3089:u8, "CCD\nEM Gain"=w3088:u16, "Readout\nRate"=w3087:u8, "Shutter\nOpenning Time"=w3086:i32, "Shutter\nClosing Time"=w3085:i32, "Vertical\nShift Speed"=w3084:u8, "Read\nMode"=w3083:u8, "Vertical\nClock Voltage"=w3082:u8, "A/D \nChannel"=w3081:u32, "Shutter\nMode"=w3080:u16, "Shutter\nTTL"=w3079:u16, "Trigger\nMode"=w3078:u16, "Frame\nTransfer"=w3058:bool, "Acquisition\nMode"=w3077:u8, "CCD \nEM Mode"=w3076:u8)
        n1693 = call-dynamic "Read AcquisitionD.vi"("error in (no error)"=w3044, "S4ACS_GUI in"=w3045) -> ("error out"=w3111:errorcluster, "Acquisition.lvclass"=w3114:refnum<class "Acquisition.lvclass">, "S4ACS_GUI out"=w3115:refnum<class "S4GUI.lvclass">)  [unwired: 7 in]
        n1694 = call-dynamic "Read Channel.vi"("error in (no error)"=w3111, "Acquisition in"=w3114) -> ("error out"=w3110:errorcluster, "Channel.lvclass"=w3112:refnum<class "Channel.lvclass">, "Acquisition out"=w3113:refnum<class "Acquisition.lvclass">)  [unwired: 7 in]
        n1695 = call-dynamic "Read Interface.vi"("error in (no error)"=w3110, "Channel in"=w3112) -> ("error out"=w3059:errorcluster, "Interface.lvclass"=w3060:refnum<class "Interface.lvclass">, "Channel out"=w3055:refnum<class "Channel.lvclass">)  [unwired: 7 in]
        n1696 = call-dynamic "Write PREV_FT.vi"("error in (no error)"=w3059, "PREV_FT"=w3058, "Interface in"=w3060) -> ("error out"=w3050:errorcluster, "Interface out"=w3056:refnum<class "Interface.lvclass">)  [unwired: 7 in]
        n1697 = call-dynamic "Read target cluster.vi"("error in (no error)"=w3050, "Channel in"=w3055) -> ("error out"=w3057:errorcluster, "target cluster"=w3054:T31, "Channel out"=w3053:refnum<class "Channel.lvclass">)  [unwired: 7 in]
        n1698 = Bundle By Name(cluster=w3054, "INITIAL_LINE"=w3095, "INITIAL_COLUMN"=w3094, "FINAL_LINE"=w3093, "FINAL_COLUMN"=w3092, "VBIN"=w3091, "HBIN"=w3090, "PREAMP"=w3089, "EM_GAIN"=w3088, "READOUT_RATE"=w3087, "SHUTTER_OPENING_TIME"=w3086, "SHUTTER_CLOSING_TIME"=w3085, "VERTICAL_SHIFT_SPEED"=w3084, "READ_MODE"=w3083, "VERTICAL_CLOCK_VOLTAGE"=w3082, "AD_CHANNEL"=w3081, "SHUTTER_MODE"=w3080, "SHUTTER_TTL"=w3079, "TRIGGER_MODE"=w3078, "FRAME_TRANSFER"=w3058, "ACQUISITION_MODE"=w3077, "EM_MODE"=w3076) -> (w3052:T31)
        n1699 = call-dynamic "Write target cluster.vi"("error in (no error)"=w3057, "target cluster"=w3052, "Channel in"=w3053) -> ("error out"=w3051:errorcluster, "Channel out"=w3049:refnum<class "Channel.lvclass">)  [unwired: 7 in]
        n1700 = Flatten To String(anything=w3052, error in (no error)=w3051) -> (data string=w3099:string, error out=w3098:errorcluster)  [unwired: 2 in, 1 out]
        n1701 = call "Write flatted cluster.vi"("error in (no error)"=w3098, "flatted cluster"=w3099, "Interface in"=w3056) -> ("error out"=w3097:errorcluster, "Interface out"=w3096:refnum<class "Interface.lvclass">)  [unwired: 7 in]
        n1702 = call-dynamic "Write Interface.vi"("error in (no error)"=w3097, "Interface.lvclass"=w3096, "Channel in"=w3049) -> ("error out"=w3071:errorcluster, "Channel out"=w3074:refnum<class "Channel.lvclass">)  [unwired: 7 in]
        n1703 = call "Write section_name.vi"("error in (no error)"=w3071, "section_name"="CCD_ACS4", "Channel in"=w3074) -> ("error out"=w3070:errorcluster, "Channel out"=w3073:refnum<class "Channel.lvclass">)  [unwired: 7 in]
        n1704 = call-dynamic "save config.vi"("error in (no error)"=w3070, "file config"="lastsaved.cfg", "Channel in"=w3073) -> ("error out"=w3069:errorcluster, "Channel out"=w3072:refnum<class "Channel.lvclass">)  [unwired: 7 in]
        n1705 = call-dynamic "Read State Machine.vi"("error in (no error)"=w3069, "Device in"=w3072) -> ("error out"=w3106:errorcluster, "State Machine.lvclass"=w3108:refnum<class "State Machine.lvclass">, "Device out"=w3109:refnum<class "Channel.lvclass">)  [unwired: 7 in]
        n1706 = call-dynamic "Write State.vi"("error in (no error)"=w3106, "State"=60, "State Machine in"=w3108) -> ("error out"=w3105:errorcluster, "State Machine out"=w3107:refnum<class "State Machine.lvclass">)  [unwired: 7 in]
        n1707 = call-dynamic "Write State Machine.vi"("error in (no error)"=w3105, "State Machine.lvclass"=w3107, "Device in"=w3109) -> ("error out"=w3102:errorcluster, "Device out"=w3103:refnum<class "Channel.lvclass">)  [unwired: 7 in]
        n1708 = call-dynamic "Write Channel.vi"("error in (no error)"=w3102, "Channel.lvclass"=w3103, "Acquisition in"=w3113) -> ("error out"=w3101:errorcluster, "Acquisition out"=w3100:refnum<class "Acquisition.lvclass">)  [unwired: 7 in]
        n1709 = call-dynamic "Write AcquisitionD.vi"("error in (no error)"=w3101, "Acquisition.lvclass"=w3100, "S4ACS_GUI in"=w3115) -> ("error out"=w3061:errorcluster, "S4ACS_GUI out"=w3062:refnum<class "S4GUI.lvclass">)  [unwired: 7 in]
        n1710 = call "Write cfg file.vi"("error in (no error)"=w3061, "cfg file"="lastsaved.cfg", "S4ACS_GUI in"=w3062) -> ("error out"=w3064:errorcluster, "S4ACS_GUI out"=w3065:refnum<class "S4GUI.lvclass">)  [unwired: 7 in]
      }
      event "Restore Default ch1": Value Change {
        n1711 = event-data() -> ()  [unwired: 1 in, 6 out]
        n1712 = call-dynamic "Read AcquisitionA.vi"("error in (no error)"=w3146, "S4ACS_GUI in"=w3147) -> ("error out"=w3142:errorcluster, "Acquisition.lvclass"=w3144:refnum<class "Acquisition.lvclass">, "S4ACS_GUI out"=w3145:refnum<class "S4GUI.lvclass">)  [unwired: 7 in]
        n1713 = call-dynamic "Read Channel.vi"("error in (no error)"=w3142, "Acquisition in"=w3144) -> ("error out"=w3129:errorcluster, "Channel.lvclass"=w3131:refnum<class "Channel.lvclass">, "Acquisition out"=w3143:refnum<class "Acquisition.lvclass">)  [unwired: 7 in]
        n1714 = call "Write section_name.vi"("error in (no error)"=w3129, "section_name"="CCD_ACS1", "Channel in"=w3131) -> ("error out"=w3128:errorcluster, "Channel out"=w3130:refnum<class "Channel.lvclass">)  [unwired: 7 in]
        n1715 = call-dynamic "load config.vi"("error in (no error)"=w3128, "cfg file name"="default.cfg", "Channel in"=w3130) -> ("error out"=w3126:errorcluster, "Channel out"=w3127:refnum<class "Channel.lvclass">)  [unwired: 7 in]
        n1716 = call-dynamic "Read State Machine.vi"("error in (no error)"=w3126, "Device in"=w3127) -> ("error out"=w3138:errorcluster, "State Machine.lvclass"=w3140:refnum<class "State Machine.lvclass">, "Device out"=w3141:refnum<class "Channel.lvclass">)  [unwired: 7 in]
        n1717 = call-dynamic "Write State.vi"("error in (no error)"=w3138, "State"=60, "State Machine in"=w3140) -> ("error out"=w3137:errorcluster, "State Machine out"=w3139:refnum<class "State Machine.lvclass">)  [unwired: 7 in]
        n1718 = call-dynamic "Write State Machine.vi"("error in (no error)"=w3137, "State Machine.lvclass"=w3139, "Device in"=w3141) -> ("error out"=w3122:errorcluster, "Device out"=w3118:refnum<class "Channel.lvclass">)  [unwired: 7 in]
        n1719 = call "Write section_name.vi"("error in (no error)"=w3122, "section_name"="CCD_ACS1", "Channel in"=w3118) -> ("error out"=w3123:errorcluster, "Channel out"=w3117:refnum<class "Channel.lvclass">)  [unwired: 7 in]
        n1720 = call-dynamic "save config.vi"("error in (no error)"=w3123, "file config"="lastsaved.cfg", "Channel in"=w3117) -> ("error out"=w3121:errorcluster, "Channel out"=w3116:refnum<class "Channel.lvclass">)  [unwired: 7 in]
        n1721 = call-dynamic "Write Channel.vi"("error in (no error)"=w3121, "Channel.lvclass"=w3116, "Acquisition in"=w3143) -> ("error out"=w3135:errorcluster, "Acquisition out"=w3134:refnum<class "Acquisition.lvclass">)  [unwired: 7 in]
        n1722 = call-dynamic "Write AcquisitionA.vi"("error in (no error)"=w3135, "Acquisition.lvclass"=w3134, "S4ACS_GUI in"=w3145) -> ("error out"=w3133:errorcluster, "S4ACS_GUI out"=w3124:refnum<class "S4GUI.lvclass">)  [unwired: 7 in]
      }
      event "Load Button": Value Change {
        (unwired) "C:\\Users\\observer\\sparc4\\s4gui\\Config" ("default name")
        n1723 = event-data() -> ()  [unwired: 1 in, 6 out]
        n1724 = String To Path(string="D:\\sparc4\\config\\s4gui" ("default name")) -> (path=w3151:path)
        n1725 = call "File Dialog"("start path"=w3151, "prompt"="Select file...", "button label"="Open", "default name"="lastsaved.cfg", "error in"=w3153, "pattern (all files)"="*.cfg") -> ("selected path"=w3150:path, "cancelled"=w3154:bool, "error out"=→"error out 2":errorcluster)  [unwired: 6 in, 1 out]
        n1726 = Strip Path(path=w3150) -> (name=w3149:string)  [unwired: 1 out]
        n1727 = case shown="False" w3154 {
          tunnel: w3161 -> [w3294 w3296]
          tunnel: [w3210 w3296] -> w3160
          tunnel: [w3208 w3295] -> w3159
          tunnel: w3153 -> [w3207 w3295]
          tunnel: w3149 -> [w3206 _]
          frame False {
            n1728 = call-dynamic "Read AcquisitionA.vi"("error in (no error)"=w3207, "S4ACS_GUI in"=w3294) -> ("error out"=w3290:errorcluster, "Acquisition.lvclass"=w3292:refnum<class "Acquisition.lvclass">, "S4ACS_GUI out"=w3293:refnum<class "S4GUI.lvclass">)  [unwired: 7 in]
            n1729 = call-dynamic "Read Channel.vi"("error in (no error)"=w3290, "Acquisition in"=w3292) -> ("error out"=w3277:errorcluster, "Channel.lvclass"=w3279:refnum<class "Channel.lvclass">, "Acquisition out"=w3291:refnum<class "Acquisition.lvclass">)  [unwired: 7 in]
            n1730 = call "Write section_name.vi"("error in (no error)"=w3277, "section_name"="CCD_ACS1", "Channel in"=w3279) -> ("error out"=w3276:errorcluster, "Channel out"=w3278:refnum<class "Channel.lvclass">)  [unwired: 7 in]
            n1731 = call-dynamic "load config.vi"("error in (no error)"=w3276, "cfg file name"=w3206, "Channel in"=w3278) -> ("error out"=w3204:errorcluster, "Channel out"=w3205:refnum<class "Channel.lvclass">)  [unwired: 7 in]
            n1732 = call-dynamic "save config.vi"("error in (no error)"=w3204, "file config"="lastsaved.cfg", "Channel in"=w3205) -> ("error out"=w3186:errorcluster, "Channel out"=w3187:refnum<class "Channel.lvclass">)  [unwired: 7 in]
            n1733 = call-dynamic "Read target cluster.vi"("error in (no error)"=w3186, "Channel in"=w3187) -> ("target cluster"=w3162:T31)  [unwired: 7 in, 2 out]
